vi "GUI_TektronixDPOSimple.vi"() -> ()   [LabVIEW 2013]
uses:
  Shared/GUI_Template/GUI_master/tcp_new_data_event.ctl
  Shared/GUI_Template/GUI_master/tcp new data cluster.ctl
panel:
  in  "Cluster":T1 caption="BELLA_TEK_DSO"
  in  "STOP":bool
  in  "GUIdevice 1":string="BELLA_TEK_DSO"
  out "error IO 2":errorcluster
  in  "insert tag":bool=TRUE
  out "tcp data event":T2
  in  "UDP error message":string
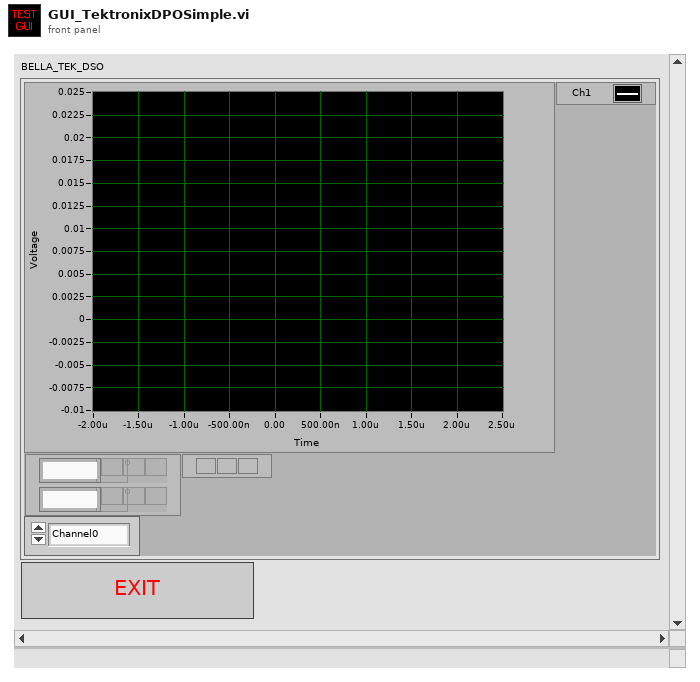
[diagram p1: front panel]
types:
  T1 = cluster{"scopeTraceGUI::1":waveform(dbl)[], "Channel::1":enum16{"Channel0", "Channel1", "Channel2", "Channel3"}}
  T2 = typedef "tcp_new_data_event.ctl" = refnum<user-event>
  T3 = typedef "tcp new data cluster.ctl" = cluster{"EventEnum":enum16{"new data", "connection status update"}, "Device name":string}
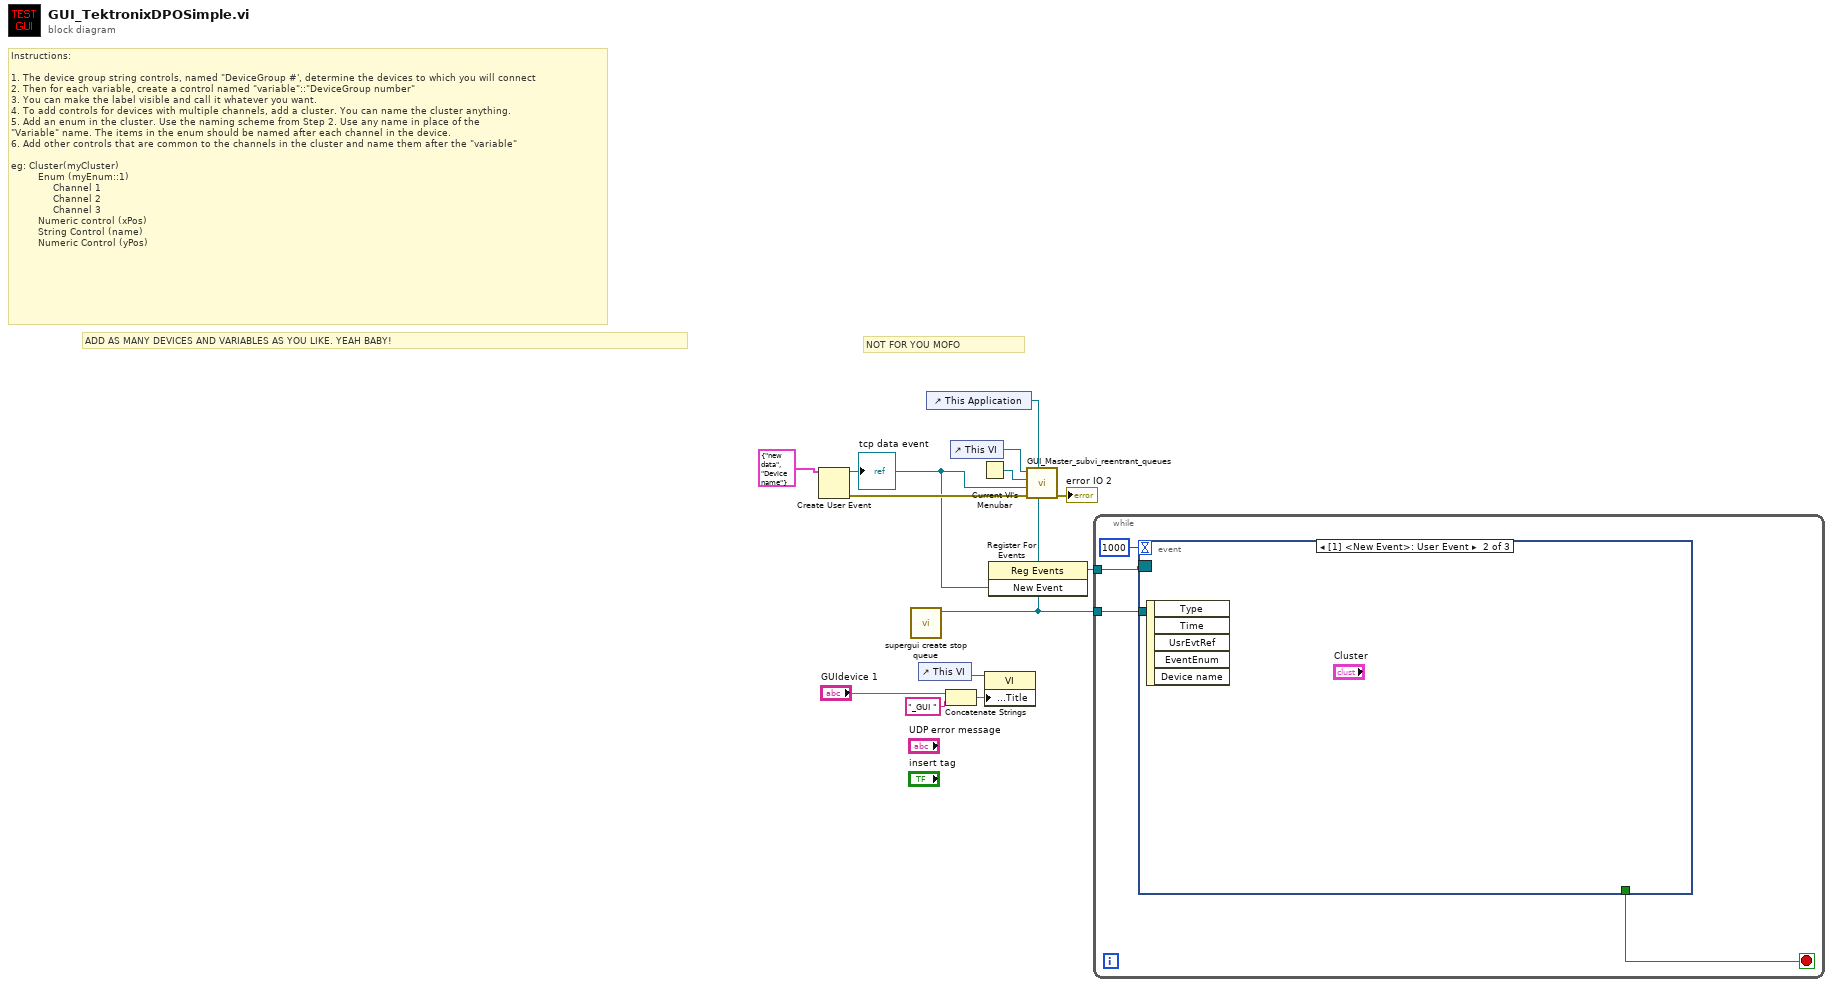
[diagram p0: block diagram]
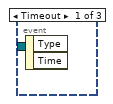
[diagram p2: hidden frame]
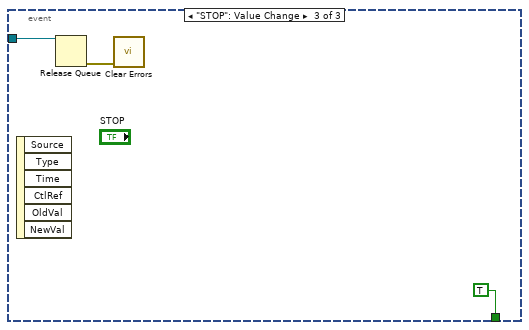
[diagram p3: hidden frame]
diagram:
  # "Instructions:\n\n1. The device group string controls, named \"DeviceGroup #', determine the devices to which you will connect\n2. Then for each variable, create a control named \"variable\"::\"DeviceGroup number\"\n3. You can make the label visible and call it whatever you want.\n4. To add controls for devices with multiple channels, add a cluster. You can name the cluster anything.\n5. Add an enum in the cluster. Use the naming scheme from Step 2. Use any name in place of the \n\"Variable\" name. The items in the enum should be named after each channel in the device. \n6. Add other controls that are common to the channels in the cluster and name them after the \"variable\"\n\neg: Cluster(myCluster)\n         Enum (myEnum::1)\n              Channel 1 \n              Channel 2\n              Channel 3\n         Numeric control (xPos)\n         String Control (name)\n         Numeric Control (yPos)"
  # "ADD AS MANY DEVICES AND VARIABLES AS YOU LIKE. YEAH BABY!"
  # "NOT FOR YOU MOFO"
  n1 = Create User Event(user event datatype=T3 {"EventEnum"=enum."new data", "Device name"="Device name"} ("New Event")) -> (user event=w7:refnum<user-event>, error out=w13:errorcluster)  [unwired: 1 in]
  "tcp data event" <- w7
  n2 = call "supergui create stop queue.vi"() -> ("STOP Queue out"=w5:refnum<queue>)  [unwired: 11 in]
  n3 = control-ref of="This VI"() -> (w4:refnum<vi>)
  n4 = control-ref of="This Application"() -> (w8:refnum<vi>)
  n5 = Concatenate Strings("GUIdevice 1", "_GUI ") -> (w3:string)
  n6 = control-ref of="This VI"() -> (w10:refnum<vi>)
  n7 = Current VI's Menubar() -> (w11:refnum<k9>)
  n8 = property class="VI"(reference=w4, "Front Panel.Title"=w3) -> ()  [unwired: 1 in, 2 out]
  n9 = register-events(w7) -> (reference out=w6:refnum<event-registration>)  [unwired: 2 in, 1 out]
  n10 = call "GUI_Master_subvi_reentrant_queues.vi"("STOP Queue in"=w5, "This Application"=w8, "error in (no error)"=w13, "tcp data event"=w7, "Caller menu reference"=w11, "Caller VI ref"=w10) -> ("error out"=→"error IO 2":errorcluster)  [unwired: 5 in]
  n11 = while {
    tunnel: w6 -> [w17]
    tunnel: w5 -> [w15]
    stop <- w14 stop-if-true
    n12 = event shown="[1] <New Event>: User Event" {
      selector: w17 -> [_ _ _]
      dyn-events: _ -> [_ _ _]
      timeout: 1000 -> [_ _ _]
      tunnel: w15 -> [_ _ w19]
      tunnel: [_ _ TRUE ("STOP")] -> w14
      event Timeout {
        n13 = event-data() -> ()  [unwired: 1 in, 2 out]
      }
      event User Event {
        n14 = event-data() -> ()  [unwired: 1 in, 5 out]
      }
      event "STOP": Value Change {
        n15 = event-data() -> ()  [unwired: 1 in, 6 out]
        n16 = Release Queue(queue=w19) -> (error out=w20:errorcluster)  [unwired: 2 in, 2 out]
        n17 = call <vilib>:"Clear Errors.vi"("error in (no error)"=w20) -> ()  [unwired: 6 in, 1 out]
      }
    }
  }
